vi "Res Array Fail check.vi"() -> ()   [LabVIEW 2013]
panel:
  out "숫자형 2":i32
  out "배열 2":bool[][](array[boolean])
  in  "정지":bool
  in  "fain number in a cycl":i16
  out "fain no":bool
  in  "duration":i32
  out "fail factor":bool
  in  "Fail No.":u16
  in  "배열":bool[](array[boolean])
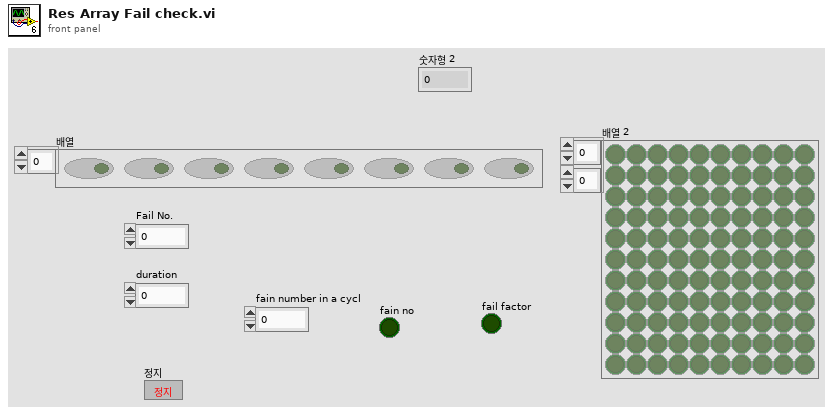
[diagram p1: front panel]
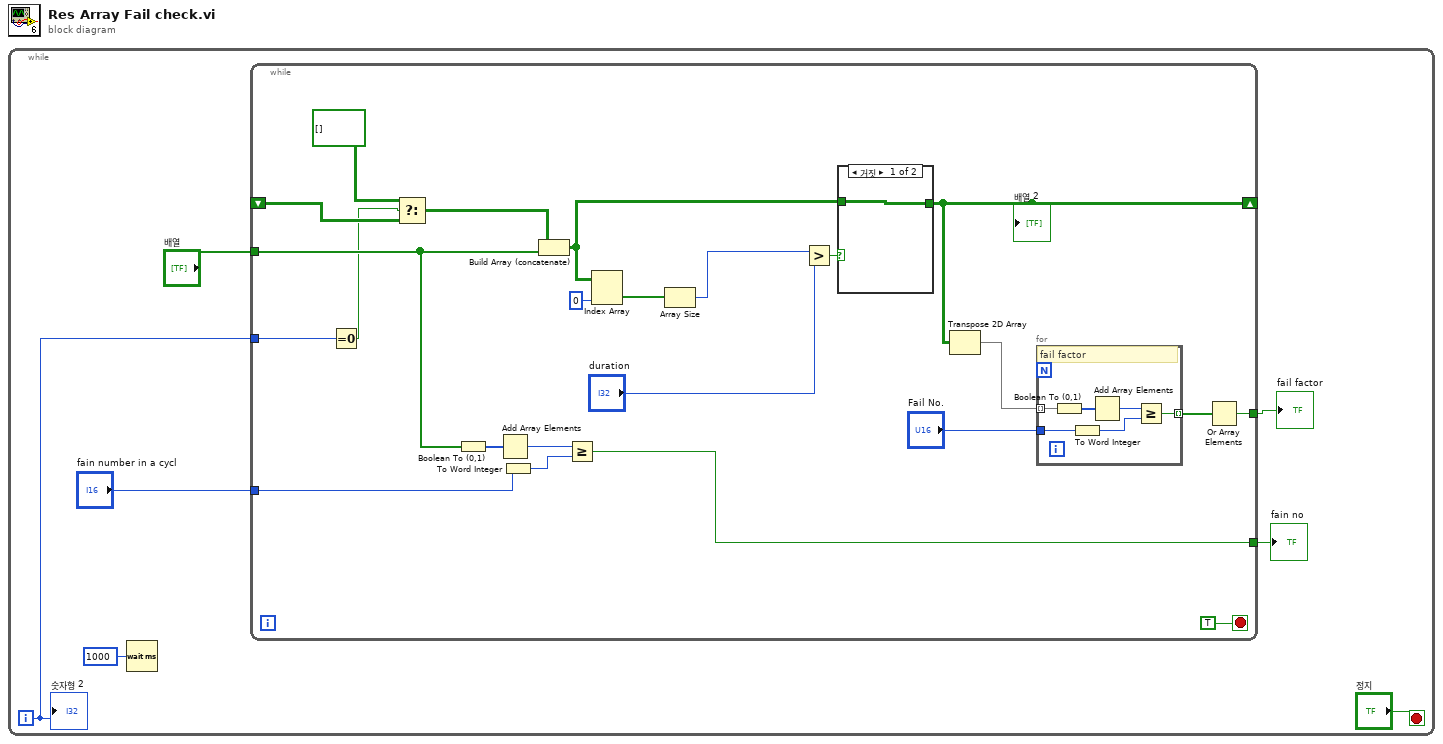
[diagram p0: block diagram]
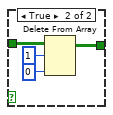
[diagram p2: hidden frame]
diagram:
  n1 = while {
    i -> [w1]
    stop <- "정지" stop-if-true
    n2 = Wait (ms)(milliseconds to wait=u32 1000 ("대기 시간(ms)")) -> ()  [unwired: 1 out]
    n3 = while {
      tunnel: [w22] -> w7
      tunnel: "배열" -> [w17]
      tunnel: [w16] -> w5
      tunnel: "fain number in a cycl" -> [w15]
      shift-right: [w12] -> _
      shift-left: _ -> [w11]
      tunnel: w1 -> [w8]
      stop <- TRUE stop-if-true
      n4 = Equal To 0?(x=w8) -> (x = 0?=w10:bool)
      n5 = Select(t=bool[][] [] ("ok/ng"), s=w10, f=w11) -> (s? t:f=w14:bool[][])
      n6 = Boolean To (0,1)(Boolean=w17) -> (0, 1=w18:i16[])
      n7 = Add Array Elements(numeric array=w18) -> (sum=w20:i16)
      n8 = To Word Integer(number=w15) -> (16bit integer=w19:i16)
      n9 = Build Array (concatenate)(w14, w17) -> (w26:bool[][])
      n10 = Greater Or Equal?(x=w20, y=w19) -> (x >= y?=w16:bool)
      n11 = Index Array(array=w26, index (col)=0 ("disabled index (col)")) -> (element=w29:bool[])  [unwired: 1 in]
      n12 = Array Size(array=w29) -> (size(s)=w27:i32)
      n13 = Greater?(x=w27, y="duration") -> (0:w28:bool)
      n14 = case shown="거짓" w28 {
        tunnel: w26 -> [w37 w41]
        tunnel: [w37 w39] -> w12
        frame False {
        }
        frame True {
          n15 = Delete From Array(array=w41, length=1, index (row)=0) -> (array with subset deleted=w39:bool[][])  [unwired: 1 in, 1 out]
        }
      }
      "배열 2" <- w12
      n16 = Transpose 2D Array(2D array=w12) -> (transposed array=w25:bool[][])
      n17 = for {
        tunnel: w25 -> [w36] mode=indexing
        tunnel: "Fail No." -> [w33]
        tunnel: [w32] -> w23 mode=indexing
        # "fail factor"
        n18 = Boolean To (0,1)(Boolean=w36) -> (0, 1=w35:i16[])
        n19 = To Word Integer(number=w33) -> (16bit integer=w31:i16)
        n20 = Add Array Elements(numeric array=w35) -> (sum=w34:i16)
        n21 = Greater Or Equal?(x=w34, y=w31) -> (x >= y?=w32:bool)
      }
      n22 = Or Array Elements(Boolean array=w23) -> (logical OR=w22:bool)
    }
    "fail factor" <- w7
    "fain no" <- w5
    "숫자형 2" <- w1
  }
